vi "CleanUp.vi"(8 "error in (no error)":errorcluster, 11 "object in":refnum<class "clear_output Message.lvclass">) -> (0 "error out":errorcluster, 3 "object out":refnum<class "clear_output Message.lvclass">)   [LabVIEW 2018, in "ClientMessaging.lvlib" / "clear_output Message.lvclass"]
uses:
  clear_output Message.lvclass
  Base Classes/Message Class/Message Class.lvclass
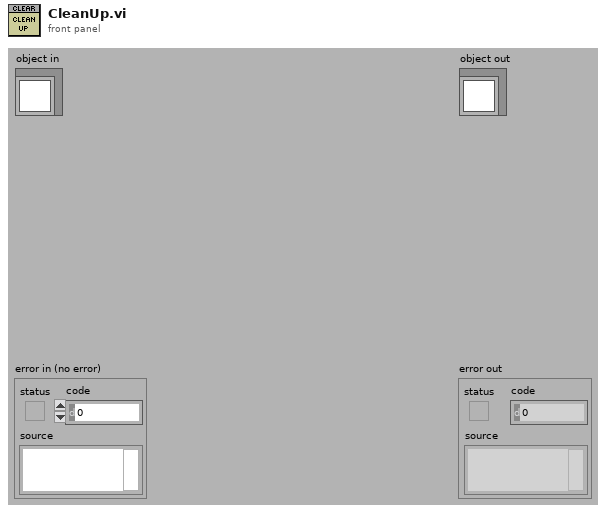
[diagram p1: front panel]
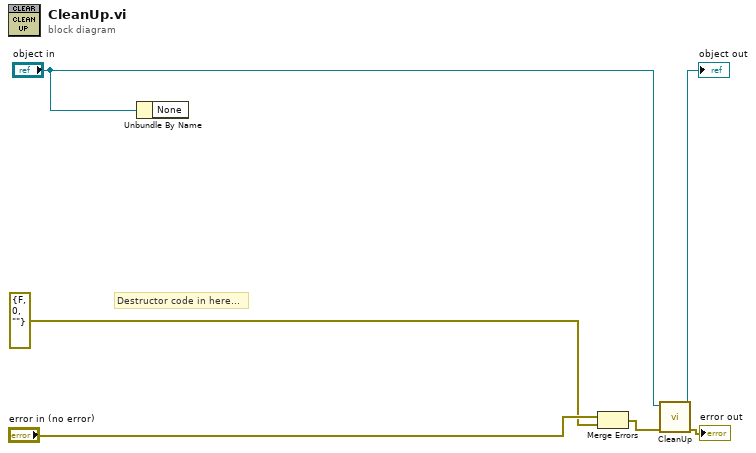
[diagram p0: block diagram]
diagram:
  # "Destructor code in here..."
  n1 = Unbundle By Name("object in") -> ()  [unwired: 1 out]
  n2 = Merge Errors("error in (no error)", errorcluster {"status"=FALSE, "code"=0, "source"=""} ("error in (no error)")) -> (w2:errorcluster)
  n3 = call-parent "CleanUp.vi"("error in (no error)"=w2, "object in"="object in") -> ("error out"=→"error out":errorcluster, "object out"=→"object out":refnum<class "clear_output Message.lvclass">)  [unwired: 8 in]
